vi "CatchAndConvertInvalidImageTypes.vi"(0 "report in":refnum<class "NI_Standard Report.lvclass">, 5 "path to image":path, 9 "image format (jpeg)":enum32{"PNG", "JPEG", "GIF"}(ring)=enum."JPEG", 11 "error in (no error)":errorcluster) -> (4 "report out":refnum<class "NI_Standard Report.lvclass">, 6 "path to image out":path, 15 "error out":errorcluster)   [LabVIEW 2020, in "NI_Standard Report.lvclass"]
uses:
  NI_Standard Report.lvclass
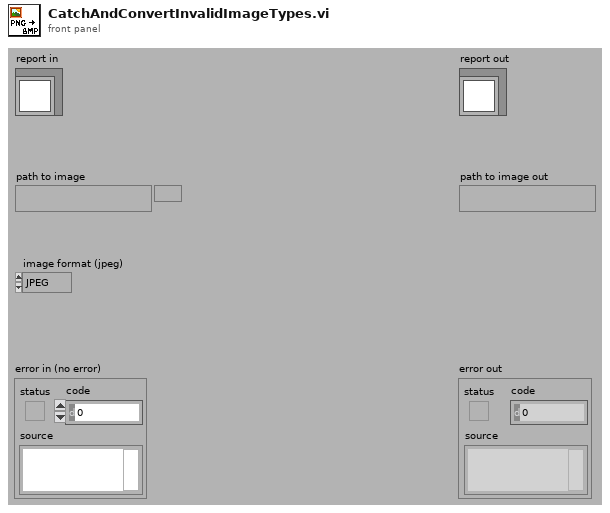
[diagram p1: front panel]
types:
  T1 = typedef "imagedata.ctl" = cluster{"image type":i32, "image depth":i32, "image":u8[], "mask":u8[], "colors":u32[], "Rectangle":cluster{"left":i16, "top":i16, "right":i16, "bottom":i16}}
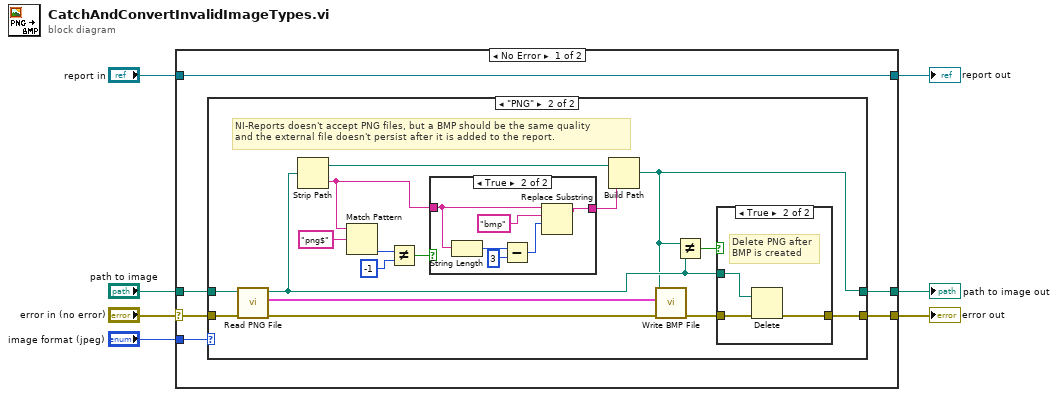
[diagram p0: block diagram]
diagram:
  n1 = case shown="No Error" "error in (no error)" {
    selector: "error in (no error)" -> [w11 w44]
    tunnel: [w10 w44] -> w6
    tunnel: [w13 w43] -> w4
    tunnel: "report in" -> [w13 w43]
    tunnel: "path to image" -> [w12 _]
    tunnel: [w9 _] -> w2
    tunnel: "image format (jpeg)" -> [w8 _]
    frame No Error {
      n2 = case shown="\"PNG\"" w8 {
        tunnel: [w14 w31] -> w10
        tunnel: w12 -> [w15 w30]
        tunnel: [w15 w16] -> w9
        tunnel: w11 -> [w14 w18]
        frame Default {
        }
        frame "PNG" {
          # "NI-Reports doesn't accept PNG files, but a BMP should be the same quality\nand the external file doesn't persist after it is added to the report."
          n3 = call "Read PNG File.vi"("error in (no error)"=w18, "path to PNG file"=w30) -> ("error out"=w28:errorcluster, "image data"=w29:T1, "path"=w17:path)  [unwired: 7 out]
          n4 = Strip Path(path=w17) -> (stripped path=w23:path, name=w24:string)
          n5 = Match Pattern(string=w24, regular expression="png$") -> (offset past match=w19:i32)  [unwired: 4 out]
          n6 = Not Equal?(x=w19, y=-1) -> (x != y?=w25:bool)
          n7 = case shown="True" w25 {
            tunnel: w24 -> [w36 w40]
            tunnel: [w36 w41] -> w22
            frame False {
            }
            frame True {
              n8 = String Length(string=w40) -> (length=w39:i32)
              n9 = Subtract(x=w39, y=3) -> (x-y=w37:i32)
              n10 = Replace Substring(3:w37, 4:"bmp" ("substring (\"\")"), 5:w40) -> (1:w41:string)  [unwired: 2 out]
            }
          }
          n11 = Build Path(base path=w23, name or relative path=w22) -> (appended path=w16:path)
          n12 = call "Write BMP File.vi"("error in (no error)"=w28, "image data"=w29, "path to BMP file"=w16) -> ("error out"=w20:errorcluster)  [unwired: 8 out]
          n13 = Not Equal?(x=w16, y=w17) -> (x != y?=w21:bool)
          n14 = case shown="True" w21 {
            tunnel: [w32 w35] -> w31
            tunnel: w17 -> [_ w34]
            tunnel: w20 -> [w32 w33]
            frame False {
            }
            frame True {
              # "Delete PNG after BMP is created"
              n15 = Delete(path (use dialog)=w34, error in=w33) -> (error out=w35:errorcluster)  [unwired: 5 out]
            }
          }
        }
      }
    }
    frame Error {
    }
  }
  "error out" <- w6
  "report out" <- w4
  "path to image out" <- w2
